vi "mp285_Move_str2xyz.vi"(0 "字符串":string) -> (1 "X轴":dbl, 2 "Y轴":dbl, 3 "Z轴":dbl)   [LabVIEW 2018]
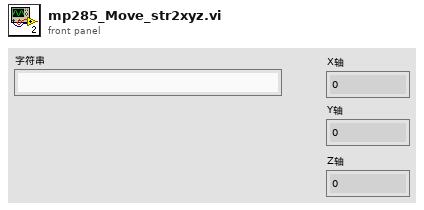
[diagram p1: front panel]
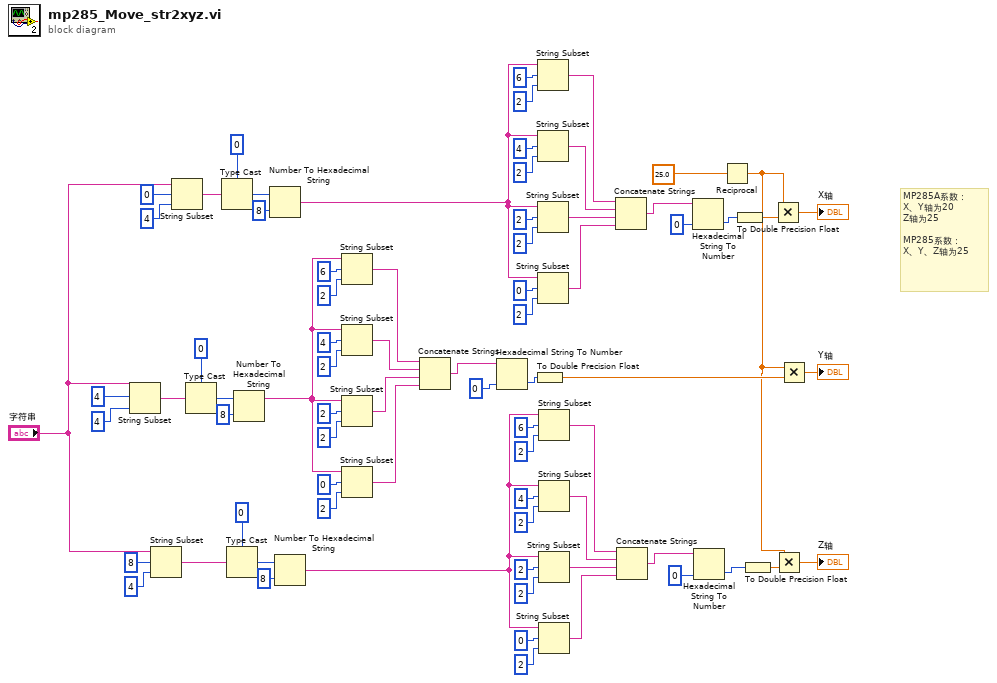
[diagram p0: block diagram]
diagram:
  # "MP285A系数：\nX、Y轴为20\nZ轴为25\n\nMP285系数：\nX、Y、Z轴为25"
  n1 = String Subset(string="字符串", offset (0)=4 ("偏移量(0)"), length (rest)=4 ("长度（剩余）")) -> (substring=w8:string)
  n2 = String Subset(string="字符串", offset (0)=8 ("偏移量(0)"), length (rest)=4 ("长度（剩余）")) -> (substring=w9:string)
  n3 = String Subset(string="字符串", offset (0)=0 ("偏移量(0)"), length (rest)=4 ("长度（剩余）")) -> (substring=w7:string)
  n4 = Type Cast(type=0, x=w8) -> (*(type *) &x=w14:i32)
  n5 = Type Cast(type=0, x=w7) -> (*(type *) &x=w17:i32)
  n6 = Type Cast(type=0, x=w9) -> (*(type *) &x=w11:i32)
  n7 = Number To Hexadecimal String(1:i16 8 ("宽度(-)"), 2:w14) -> (0:w12:string)
  n8 = Number To Hexadecimal String(1:i16 8 ("宽度(-)"), 2:w17) -> (0:w15:string)
  n9 = Number To Hexadecimal String(1:i16 8 ("宽度(-)"), 2:w11) -> (0:w5:string)
  n10 = String Subset(string=w12, offset (0)=6 ("偏移量(0)"), length (rest)=2 ("长度（剩余）")) -> (substring=w51:string)
  n11 = String Subset(string=w12, offset (0)=4 ("偏移量(0)"), length (rest)=2 ("长度（剩余）")) -> (substring=w52:string)
  n12 = String Subset(string=w12, offset (0)=2 ("偏移量(0)"), length (rest)=2 ("长度（剩余）")) -> (substring=w53:string)
  n13 = String Subset(string=w12, offset (0)=0 ("偏移量(0)"), length (rest)=2 ("长度（剩余）")) -> (substring=w54:string)
  n14 = Concatenate Strings(w51, w52, w53, w54) -> (w62:string)
  n15 = Hexadecimal String To Number(string=w62, default (0uL)=0 ("默认(0 U32)")) -> (number=w34:i32)  [unwired: 1 in, 1 out]
  n16 = To Double Precision Float(number=w34) -> (double precision float=w31:dbl)
  n17 = String Subset(string=w15, offset (0)=6 ("偏移量(0)"), length (rest)=2 ("长度（剩余）")) -> (substring=w73:string)
  n18 = String Subset(string=w15, offset (0)=4 ("偏移量(0)"), length (rest)=2 ("长度（剩余）")) -> (substring=w72:string)
  n19 = String Subset(string=w15, offset (0)=2 ("偏移量(0)"), length (rest)=2 ("长度（剩余）")) -> (substring=w71:string)
  n20 = String Subset(string=w15, offset (0)=0 ("偏移量(0)"), length (rest)=2 ("长度（剩余）")) -> (substring=w70:string)
  n21 = String Subset(string=w5, offset (0)=6 ("偏移量(0)"), length (rest)=2 ("长度（剩余）")) -> (substring=w46:string)
  n22 = String Subset(string=w5, offset (0)=4 ("偏移量(0)"), length (rest)=2 ("长度（剩余）")) -> (substring=w45:string)
  n23 = String Subset(string=w5, offset (0)=2 ("偏移量(0)"), length (rest)=2 ("长度（剩余）")) -> (substring=w44:string)
  n24 = String Subset(string=w5, offset (0)=0 ("偏移量(0)"), length (rest)=2 ("长度（剩余）")) -> (substring=w43:string)
  n25 = Concatenate Strings(w73, w72, w71, w70) -> (w20:string)
  n26 = Concatenate Strings(w46, w45, w44, w43) -> (w35:string)
  n27 = Hexadecimal String To Number(string=w20, default (0uL)=0 ("默认(0 U32)")) -> (number=w18:i32)  [unwired: 1 in, 1 out]
  n28 = Hexadecimal String To Number(string=w35, default (0uL)=0 ("默认(0 U32)")) -> (number=w33:i32)  [unwired: 1 in, 1 out]
  n29 = Reciprocal(x=25.0) -> (1/x=w6:dbl)
  n30 = To Double Precision Float(number=w18) -> (double precision float=w19:dbl)
  n31 = To Double Precision Float(number=w33) -> (double precision float=w32:dbl)
  n32 = Multiply(x=w6, y=w19) -> (x*y=→"X轴":dbl)
  n33 = Multiply(x=w6, y=w32) -> (x*y=→"Z轴":dbl)
  n34 = Multiply(x=w6, y=w31) -> (x*y=→"Y轴":dbl)
